vi "video.vi"() -> ()   [LabVIEW 2017]
uses:
  <vilib>/userdefined/High Color/IMAQdx.ctl
  <vilib>/myRIO/Instrument Drivers/Onboard IO/PWM/typedefs/PWM Reference.ctl
  <vilib>/myRIO/Common/Instrument Driver Framework/Utilities/typedefs/myRIO Generic Hardware Reference.ctl
  <vilib>/myRIO/Common/Instrument Driver Framework/Utilities/typedefs/Hardware Version Enum.ctl
  <vilib>/myRIO/Common/Instrument Driver Framework/Utilities/typedefs/myRIO v1.0 Reference.ctl
  <vilib>/myRIO/Common/Instrument Driver Framework/Utilities/typedefs/Generic FPGA Reference.ctl
  <vilib>/myRIO/Common/Instrument Driver Framework/myRIO v1.0/PWM/typedefs/PWM Channels Enum.ctl
  <vilib>/myRIO/Instrument Drivers/Onboard IO/PWM/typedefs/PWM Configuration.ctl
  <vilib>/userdefined/High Color/nirio_resource_hc.ctl
  <vilib>/myRIO/Common/Instrument Driver Framework/Utilities/vis/Is FPGA Ref Available.vi
  <vilib>/myRIO/Common/Instrument Driver Framework/myRIO v1.0/PWM/vis/myRIO v1.1 Open PWM.vi
  <vilib>/myRIO/Instrument Drivers/Onboard IO/PWM/vis/Set Duty Cycle and Frequency.vi
  <vilib>/myRIO/Common/Instrument Driver Framework/Utilities/vis/Validate Channels.vi
  <vilib>/myRIO/Common/Instrument Driver Framework/myRIO v1.0/PWM/vis/myRIO v1.0 Reserve PWM.vi
  <vilib>/myRIO/Common/Instrument Driver Framework/myRIO v1.0/PWM/vis/myRIO v1.0 Build MUX Configuration PWM.vi
  <vilib>/myRIO/Common/Instrument Driver Framework/myRIO v1.0/Resource Manager/vis/myRIO v1.0 Reserve Channel List.vi
  <vilib>/myRIO/Common/Instrument Driver Framework/myRIO v1.0/Resource Manager/vis/myRIO v1.0 Create Configuration List.vi
  <vilib>/myRIO/Common/Instrument Driver Framework/myRIO v1.0/Resource Manager/vis/myRIO v1.0 Reserve Channel.vi
  <vilib>/myRIO/Common/Instrument Driver Framework/myRIO v1.0/Resource Manager/vis/myRIO v1.0 Unreserve Channel.vi
  <vilib>/myRIO/Common/Instrument Driver Framework/myRIO v1.0/Resource Manager/vis/myRIO v1.0 Build Mutex Name.vi
  <vilib>/Utility/VariantDataType/GetNumericInfo.vi
  <vilib>/Utility/error.llb/Error Cluster From Error Code.vi
  <vilib>/myRIO/Common/Instrument Driver Framework/myRIO v1.0/myRIO v1.1 Open.vi
  <vilib>/myRIO/Common/Instrument Driver Framework/Utilities/vis/IO Manager.vi
  <vilib>/myRIO/Common/Instrument Driver Framework/Utilities/vis/Configuration Manager.vi
  <vilib>/myRIO/Common/Instrument Driver Framework/myRIO v1.0/Resource Manager/vis/myRIO v1.0 Configure IO.vi
  <vilib>/myRIO/Common/Instrument Driver Framework/myRIO v1.0/myRIO v1.0 Close.vi
  <vilib>/myRIO/Common/Instrument Driver Framework/myRIO v1.0/PWM/vis/myRIO v1.0 Write PWM.vi
  <vilib>/myRIO/Express VI/Onboard IO/PWM/PWM Express VI.xnode
  <vilib>/myRIO/Instrument Drivers/Onboard IO/PWM/vis/myRIO PWM Open.xnode
  <vilib>/vision/driver/NI_Vision_Acquisition_Software.lvlib
  <vilib>/myRIO/Instrument Drivers/Onboard IO/PWM/PWM.lvlib
panel:
  out "X":sgl
  in  "stop 2":bool
  out "peh":i32
  out "stop":i32
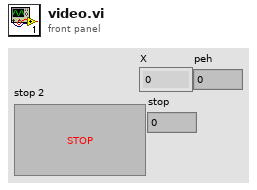
[diagram p1: front panel]
types:
  T1 = typedef "IMAQdx.ctl" = refnum<k21>
  T2 = typedef "IMAQ Image.ctl" = refnum<image>
  T3 = typedef "PWM.lvlib/PWM Reference.ctl" = cluster{"myRIO Reference":T4, "PWM Channels Enum":T8, "PWM Configuration":T9}
  T4 = typedef "myRIO Generic Hardware Reference.ctl" = cluster{"myRIO Model":T5, "myRIO Hardware Reference":T6}
  T5 = typedef "Hardware Version Enum.ctl" = enum16{"Unknown", "myRIO-1900", "myRIO-1950", "roboRIO", "NI ELVIS RIO CM"}
  T6 = typedef "myRIO v1.0 Reference.ctl" = cluster{"Generic FPGA Reference":T7, "Allow multiple opens":bool}
  T7 = typedef "Generic FPGA Reference.ctl" = refnum<k20>
  T8 = typedef "PWM Channels Enum.ctl" = enum16{"Not Connected", "C/PWM0", "C/PWM1", "A/PWM0", "A/PWM1", "A/PWM2", "B/PWM0", "B/PWM1", "B/PWM2", "PWM/PWM0", "PWM/PWM1", "PWM/PWM2", "PWM/PWM3", "PWM/PWM4", "PWM/PWM5", "PWM/PWM6", "PWM/PWM7", "PWM/PWM8", "PWM/PWM9"}
  T9 = typedef "PWM.lvlib/PWM Configuration.ctl" = cluster{"Frequency":dbl, "Duty Cycle":dbl}
  T10 = typedef "nirio_resource_hc.ctl" = tag
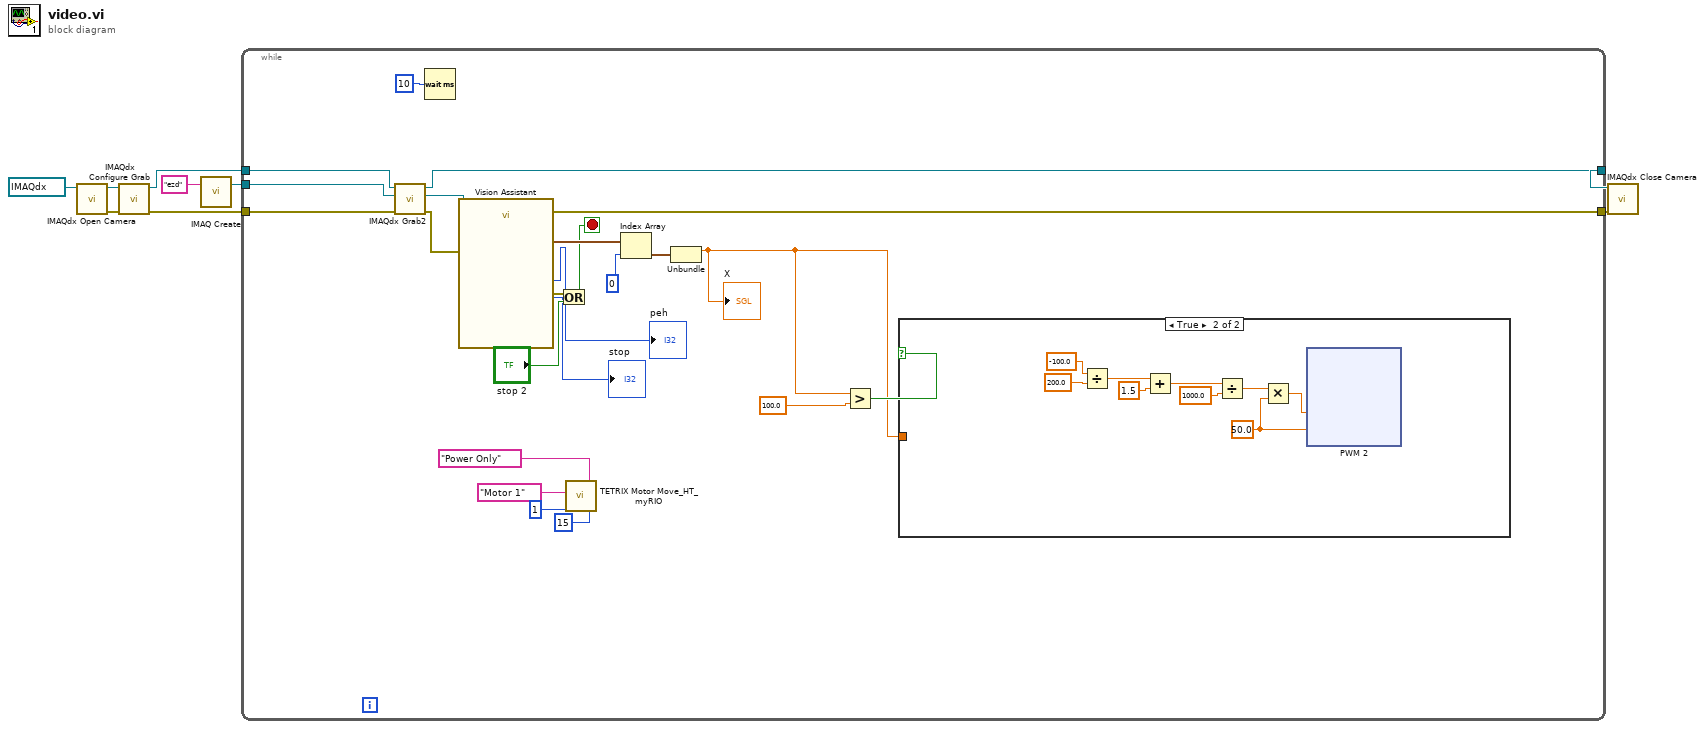
[diagram p0: block diagram]
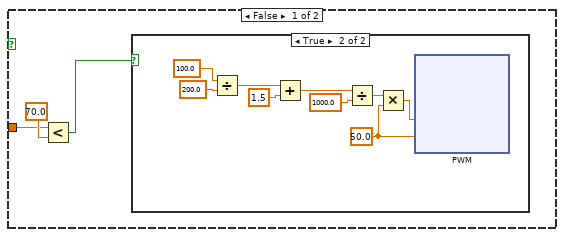
[diagram p2: hidden frame]
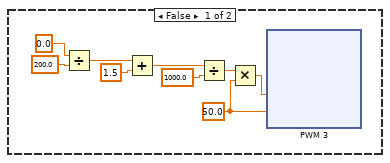
[diagram p3: hidden frame]
diagram:
  n1 = call <vilib>:"IMAQdx Open Camera.vi"("Session In"=T1 "cam0") -> ("error out"=w6:errorcluster, "Session Out"=w7:T1)  [unwired: 9 in]
  n2 = call <vilib>:"IMAQdx Configure Grab.vi"("error in"=w6, "Session In"=w7) -> ("error out"=w5:errorcluster, "Session Out"=w8:T1)  [unwired: 8 in]
  n3 = call "IMAQ Create"("Image Name"="ezd") -> ("New Image"=w9:T2)  [unwired: 4 in, 1 out]
  n4 = while {
    tunnel: w5 -> [w26]
    tunnel: w9 -> [w25]
    tunnel: w8 -> [w24]
    tunnel: [w23] -> w3
    tunnel: [w19] -> w4
    stop <- w18 stop-if-true
    n5 = call <vilib>:"IMAQdx Grab2.vi"("error in"=w26, "Image In"=w25, "Session In"=w24) -> ("error out"=w28:errorcluster, "Image Out"=w27:T2, "Session Out"=w23:T1)  [unwired: 5 in, 1 out]
    n6 = Wait (ms)(milliseconds to wait=u32 10) -> ()  [unwired: 1 out]
    n7 = call "Vision Assistant"("Image In"=w27, "error in"=w28) -> ("Edges Coordinates (Edge Detector 1)"=w31:cluster{"X":sgl, "Y":sgl}[], "Number of Matches (Color Location 2)"=→"peh":i32, "Number of Matches (Color Location 1)"=→"stop":i32, "error out"=w19:errorcluster)  [unwired: 20 in, 2 out]
    n8 = Or(x=w19, y="stop 2") -> (x .or. y?=w18:bool)
    n9 = call <vilib>:"TETRIX Motor Move_HT_myRIO.vi"("Power (-100 to 100)\n0 = Stop/Brake\n-128 = Stop/Coast"=i8 15 ("Power (-100 to 100)\n0 = Stop/Brake\n-128 = Stop/Coast"), "Control Mode"="Power Only", "Controller Daisy Chain Position: 1 - 4"=u8 1, "Select Channel"="Motor 1") -> ()  [unwired: 3 in, 1 out]
    n10 = Index Array(array=w31, index=0) -> (element=w30:cluster{"X":sgl, "Y":sgl})
    n11 = Unbundle(w30) -> ("X"=w14:sgl)  [unwired: 1 out]
    "X" <- w14
    n12 = Greater?(x=w14, y=sgl 100.0) -> (0:w15:bool)
    n13 = case shown="True" w15 {
      tunnel: w14 -> [w33 _]
      frame False {
        n14 = Less?(x=w33, y=sgl 70.0) -> (x < y?=w32:bool)
        n15 = case shown="True" w32 {
          frame False {
            w39 = 50.0 ("Frequency [Hz]")
            n16 = Divide(x=0.0, y=200.0) -> (x/y=w42:dbl)
            n17 = Add(x=w42, y=1.5) -> (x+y=w41:dbl)
            n18 = Divide(x=w41, y=1000.0) -> (x/y=w40:dbl)
            n19 = Multiply(x=w40, y=w39) -> (x*y=w43:dbl)
            n20 = xnode "PWM 3"("Duty Cycle"=w43, "Frequency [Hz]"=w39) -> ()  [unwired: 1 in, 1 out]
          }
          frame True {
            w83 = 50.0 ("Frequency [Hz]")
            n21 = Divide(x=100.0, y=200.0) -> (x/y=w86:dbl)
            n22 = Add(x=w86, y=1.5) -> (x+y=w85:dbl)
            n23 = Divide(x=w85, y=1000.0) -> (x/y=w84:dbl)
            n24 = Multiply(x=w84, y=w83) -> (x*y=w87:dbl)
            n25 = xnode "PWM"("Duty Cycle"=w87, "Frequency [Hz]"=w83) -> ()  [unwired: 1 in, 1 out]
          }
        }
      }
      frame True {
        w127 = 50.0 ("Frequency [Hz]")
        n26 = Divide(x=-100.0, y=200.0) -> (x/y=w130:dbl)
        n27 = Add(x=w130, y=1.5) -> (x+y=w129:dbl)
        n28 = Divide(x=w129, y=1000.0) -> (x/y=w128:dbl)
        n29 = Multiply(x=w128, y=w127) -> (x*y=w131:dbl)
        n30 = xnode "PWM 2"("Duty Cycle"=w131, "Frequency [Hz]"=w127) -> ()  [unwired: 1 in, 1 out]
      }
    }
  }
  n31 = call <vilib>:"IMAQdx Close Camera.vi"("error in"=w4, "Session In"=w3) -> ()  [unwired: 9 in, 1 out]
